vi "Connect.vi"(8 "error in (no error)":errorcluster, 9 "timeout":i32=-1, 11 "TCP Stream Initiator in":refnum<class "TCP Stream Initiator.lvclass">) -> (0 "error out":errorcluster, 3 "TCP Stream Initiator out":refnum<class "TCP Stream Initiator.lvclass">)   [LabVIEW 2020, in "TCP Stream Initiator.lvclass"]
doc: "This method initiates a connection between a TCP/IP Initiator/Listener pair."
uses:
  TCP Stream Initiator.lvclass
  TCP Stream/TCP Stream.lvclass
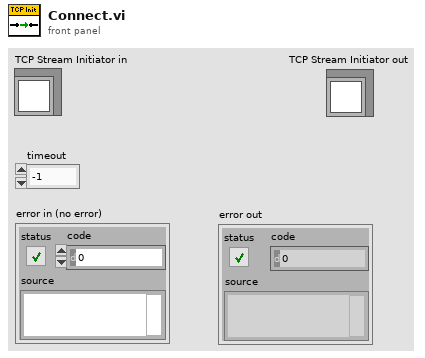
[diagram p1: front panel]
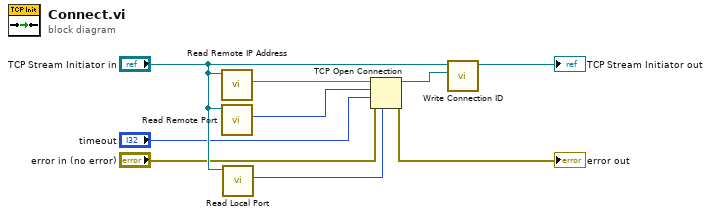
[diagram p0: block diagram]
diagram:
  n1 = call "Read Remote IP Address.vi"("TCP Stream in"="TCP Stream Initiator in") -> ("Remote IP"=w3:string)  [unwired: 10 in]
  n2 = call "Read Remote Port.vi"("TCP Stream in"="TCP Stream Initiator in") -> ("remote port"=w2:u16)  [unwired: 10 in]
  n3 = call "Read Local Port.vi"("TCP Stream in"="TCP Stream Initiator in") -> ("local port"=w1:u16)  [unwired: 10 in]
  n4 = TCP Open Connection(address=w3, remote port or service name=w2, timeout ms (60000)="timeout", local port=w1, error in (no error)="error in (no error)") -> (connection ID=w4:refnum<k5>, error out=→"error out":errorcluster)
  n5 = call "Write Connection ID.vi"("connection ID"=w4, "TCP Stream in"="TCP Stream Initiator in") -> ("TCP Stream out"=→"TCP Stream Initiator out":refnum<class "TCP Stream Initiator.lvclass">)  [unwired: 9 in]
